vi "Test - Thermal Chamber Controller_DQMH - Update Heater State 1-teardown.vi"(7 "test case ID":string, 8 "error in (no error)":errorcluster) -> (3 "result":bool)   [LabVIEW 2018]
uses:
  Libraries/Thermal Chamber Response Simulator/Thermal Chamber Response Simulator.lvlib
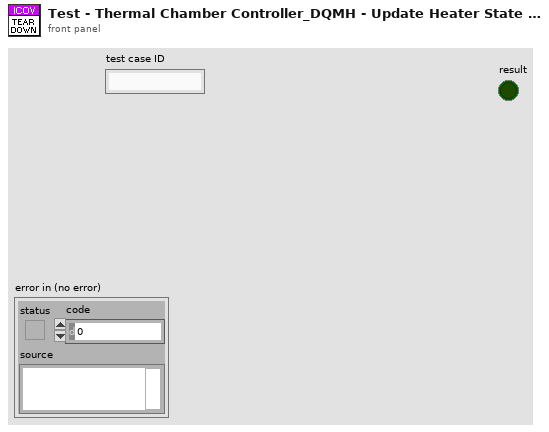
[diagram p1: front panel]
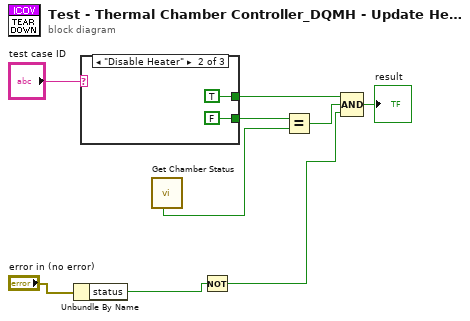
[diagram p0: block diagram]
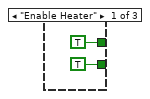
[diagram p2: hidden frame]
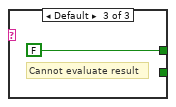
[diagram p3: hidden frame]
diagram:
  n1 = Unbundle By Name("error in (no error)") -> ("status"=w2:bool)
  n2 = case shown="\"Disable Heater\"" "test case ID" {
    tunnel: [TRUE ("Heater State") FALSE ("Heater State") _] -> w6
    tunnel: [TRUE ("value") TRUE ("value") FALSE ("value")] -> w4
    frame "Enable Heater" {
    }
    frame "Disable Heater" {
    }
    frame Default {
      # "Cannot evaluate result"
    }
  }
  n3 = call "Get Chamber Status.vi"() -> ("Heater State"=w5:bool)  [unwired: 6 in, 5 out]
  n4 = Not(x=w2) -> (.not. x?=w1:bool)
  n5 = Equal?(x=w6, y=w5) -> (x = y?=w8:bool)
  n6 = Compound Arithmetic op=AND(w4, w8, w1) -> (→"result":bool)
